vi "VI Tree - boolean__ogtk.vi"   [LabVIEW 2014]
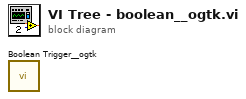
[diagram p0: block diagram]
diagram:
  n1 = call <userlib>:"Boolean Trigger__ogtk.vi"() -> ()  [unwired: 2 in, 2 out]
